vi "1d.vi"(6 "data in":T2={"Total counts"=0, "cps"=0.0, "live time"=0.0, "pulser"=0.0, "rare counts"=0.0, "other counts"=0.0, "total run time(sec)"=0.0, "adjusted run time(sec)"=0.0, "17O average"=1.0, "17O current"=1.0}, 8 "error in":errorcluster, 9 "1d state control":T3) -> (2 "MCA Histograms":u32[](graph), 4 "data out":T2={"Total counts"=0, "cps"=0.0, "live time"=0.0, "pulser"=0.0, "rare counts"=0.0, "other counts"=0.0, "total run time(sec)"=0.0, "adjusted run time(sec)"=0.0, "17O average"=1.0, "17O current"=1.0})   [LabVIEW 2016]
doc: "uses gated region to gather and parse 1d data"
uses:
  controls/1d/1d state event control.ctl
  spectrum/controls/count control.ctl
  Drivers/Pixie4DLL.dll
panel:
  out "Run time [s]":dbl
  out "number of events":dbl
  out "run data output":T1
  out "time":dbl
  out "counts":dbl
  in  "time for each slice(ms)":i32=100
  out "cps (slice)":dbl
  out "Pixie4DLL calls error":errorcluster
  out "run time":sgl
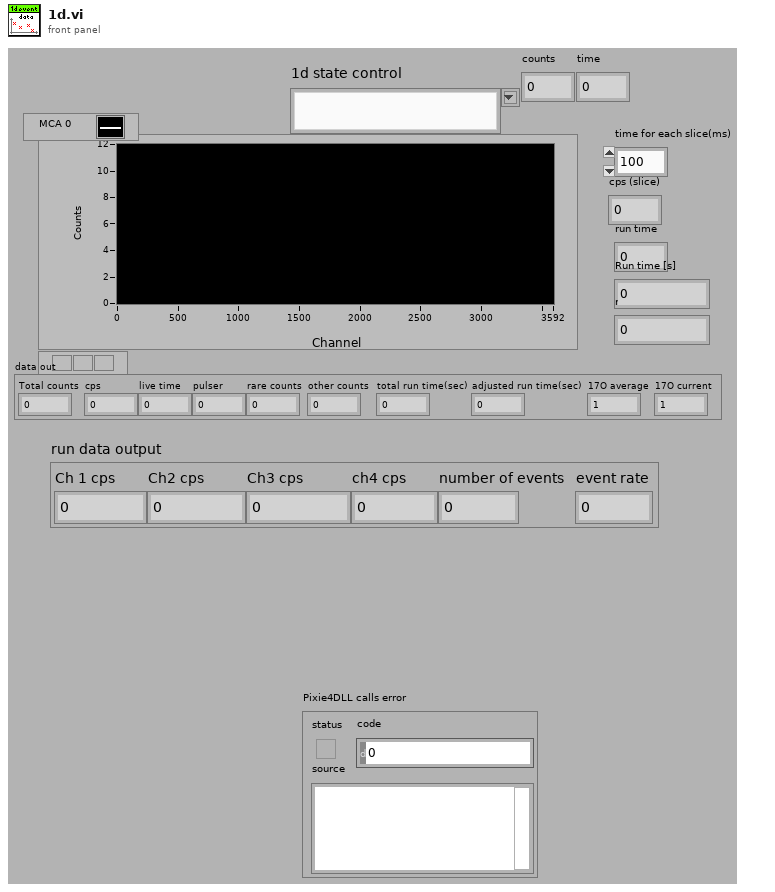
[diagram p1: front panel]
types:
  T1 = cluster{"Ch 1 cps":dbl, "Ch2 cps":dbl, "Ch3 cps":dbl, "ch4 cps":dbl, "number of events":dbl, "event rate":dbl}
  T2 = typedef "count control.ctl" = cluster{"Total counts":u32, "cps":dbl, "live time":dbl, "pulser":dbl, "rare counts":dbl, "other counts":dbl, "total run time(sec)":dbl, "adjusted run time(sec)":dbl, "17O average":dbl, "17O current":dbl}
  T3 = typedef "1d state event control.ctl" = string
  T4 = cluster{"input count rate 0":dbl, "input count rate 1":dbl, "input count rate 2":dbl, "input count rate 3":dbl, "number of events":dbl, "event rate":dbl}
  T5 = typedef "LVPoint32TypeDef.ctl" = cluster{"Horizontal":i32, "Vertical":i32}
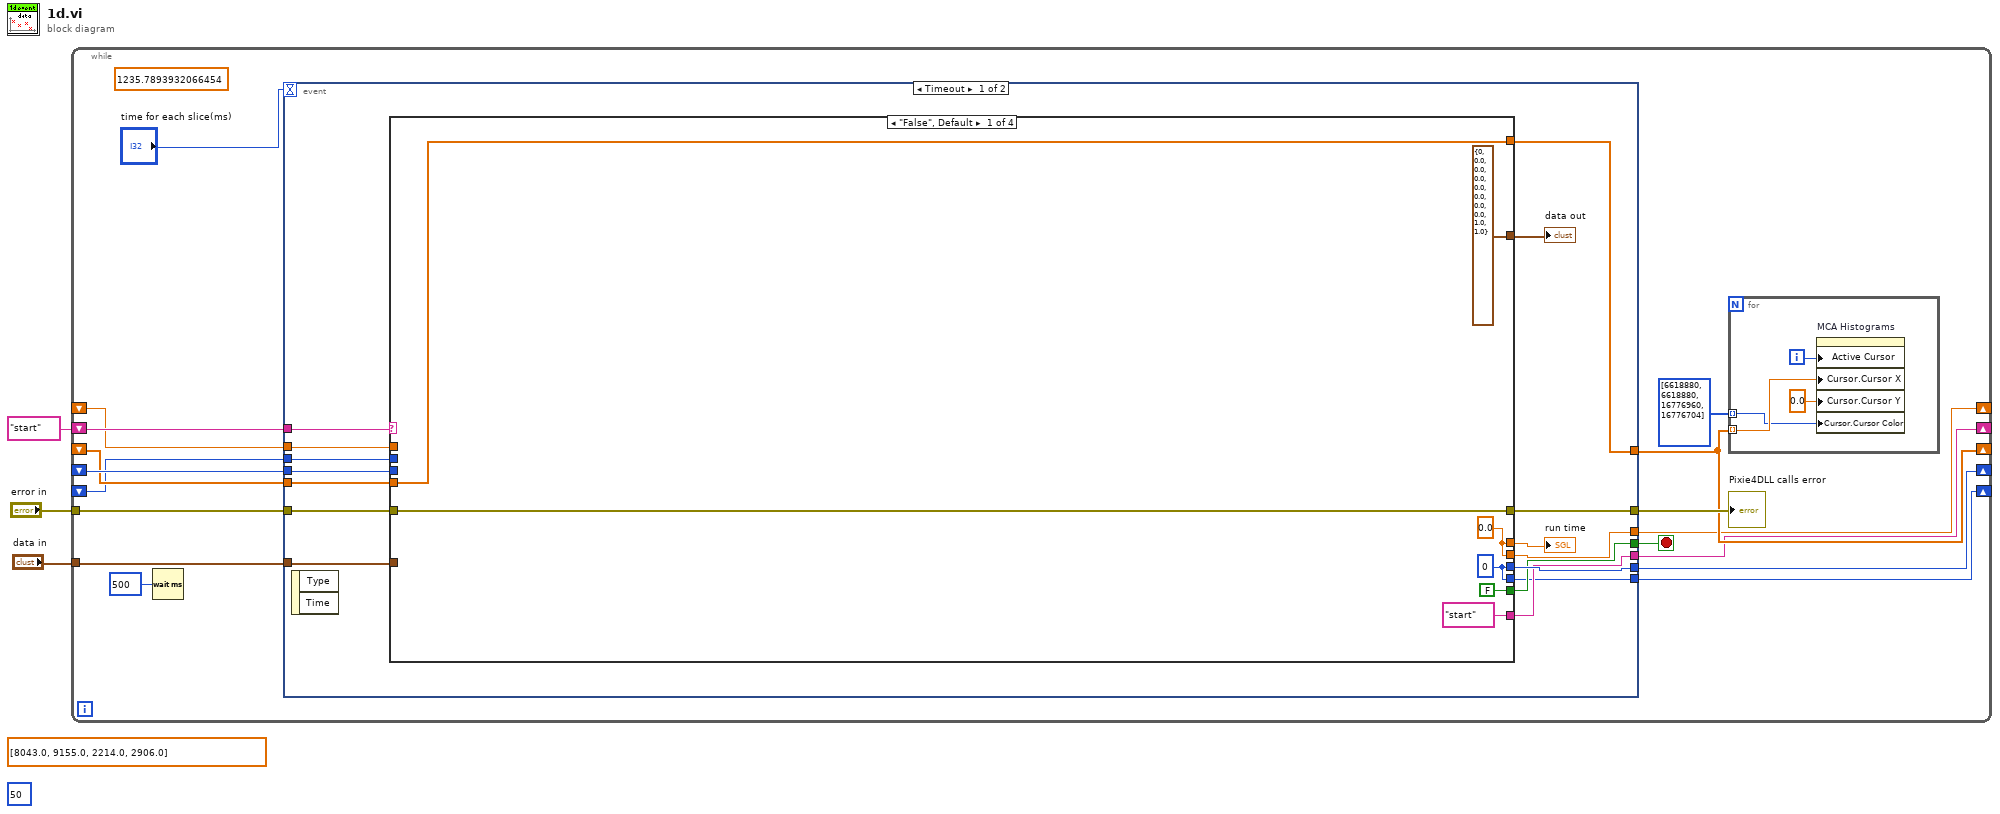
[diagram p0: block diagram]
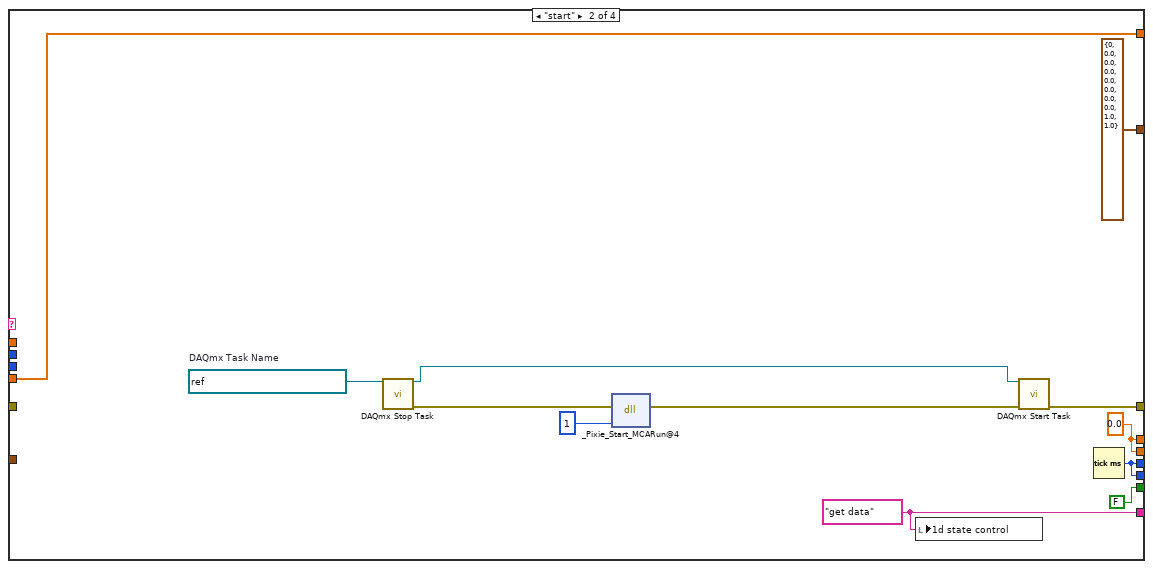
[diagram p2: hidden frame]
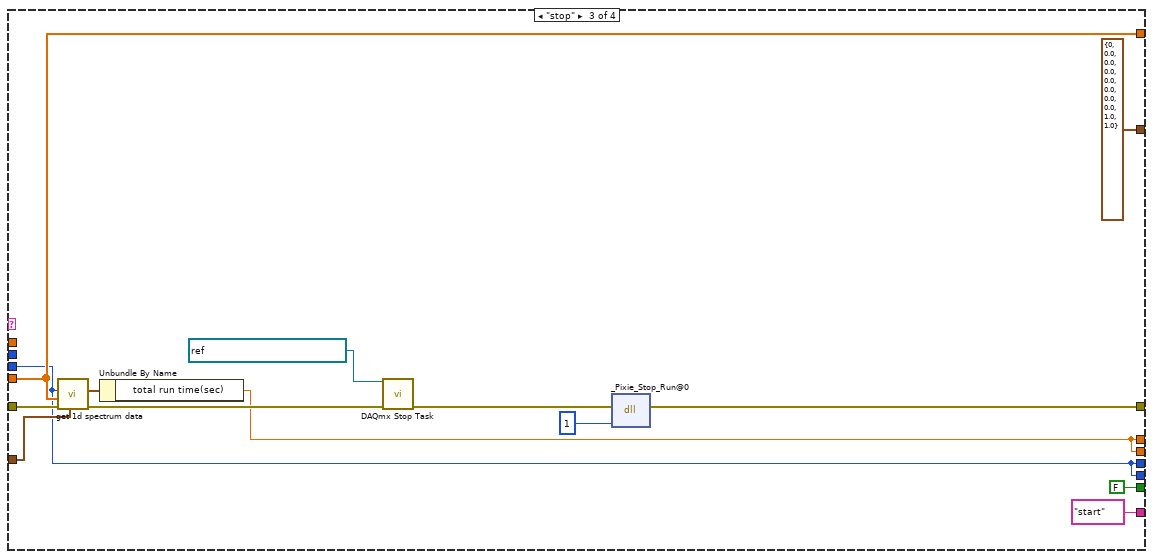
[diagram p3: hidden frame]
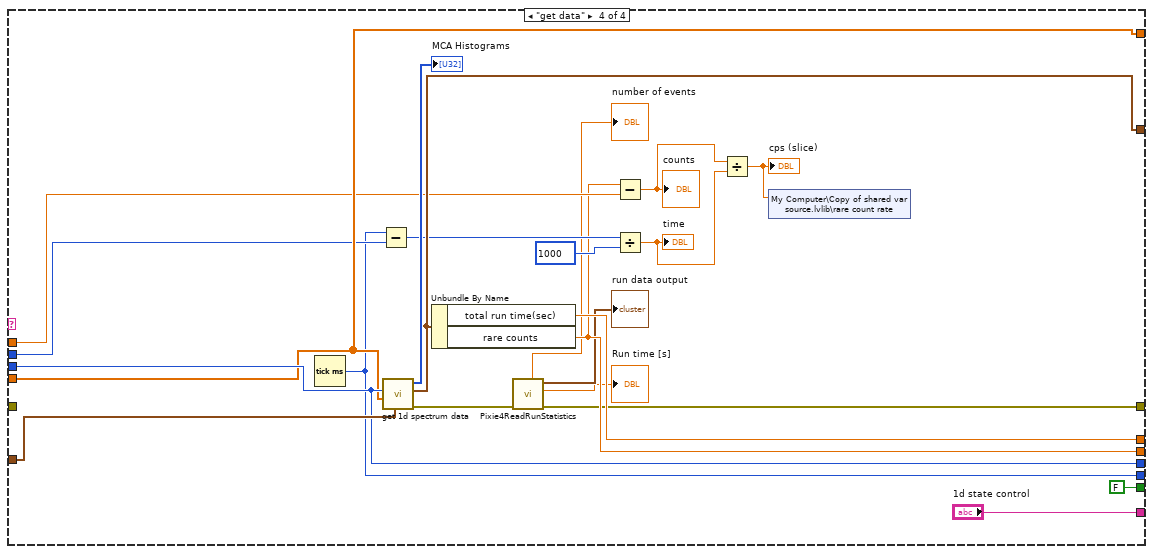
[diagram p4: hidden frame]
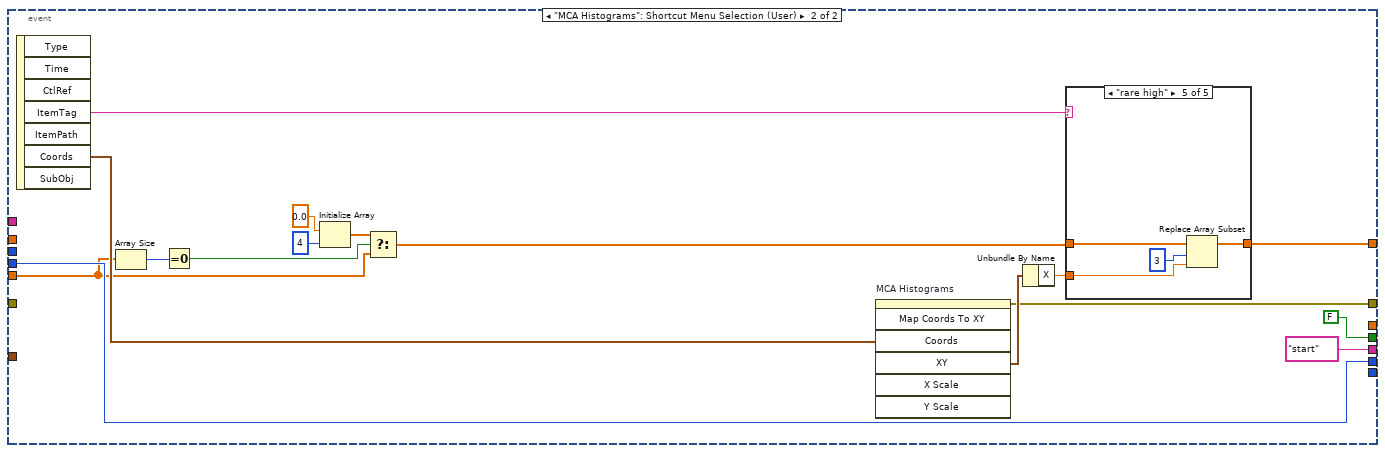
[diagram p5: hidden frame]
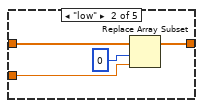
[diagram p7: hidden frame]
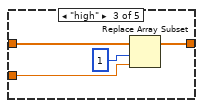
[diagram p8: hidden frame]
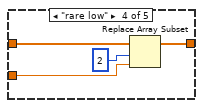
[diagram p9: hidden frame]
diagram:
  (unwired) dbl[] [8043.0, 9155.0, 2214.0, 2906.0] ("Array 2")
  (unwired) 50
  n1 = while {
    tunnel: "error in" -> [w18]
    tunnel: "data in" -> [w17]
    shift-right: [w16] -> _
    shift-left: _ -> [w20]
    shift-right: [w11] -> _
    shift-left: _ -> [w19]
    shift-right: [w8] -> _
    shift-left: T3 "start" ("1d state control") -> [w14]
    shift-right: [w7] -> _
    shift-left: _ -> [w6]
    shift-right: [w5] -> _
    shift-left: _ -> [w4]
    stop <- w13 stop-if-true
    (unwired) 1235.7893932066454 ("element")
    n2 = Wait (ms)(milliseconds to wait=u32 500) -> ()  [unwired: 1 out]
    n3 = event shown="[0] Timeout" {
      selector: _ -> [_ _]
      dyn-events: _ -> [_ _]
      timeout: "time for each slice(ms)" -> [_ _]
      tunnel: w20 -> [w40 w111]
      tunnel: w19 -> [w38 w100]
      tunnel: w18 -> [w37 _]
      tunnel: w17 -> [w36 _]
      tunnel: [w35 w111] -> w16
      tunnel: [w34 w106] -> w11
      tunnel: w14 -> [w33 _]
      tunnel: [w30 FALSE ("stop")] -> w13
      tunnel: [w32 w97] -> w12
      tunnel: [w29 T3 "start" ("1d state control")] -> w8
      tunnel: [w28 _] -> w7
      tunnel: w6 -> [w27 _]
      tunnel: [w26 _] -> w5
      tunnel: w4 -> [w25 _]
      event Timeout {
        n4 = event-data() -> ()  [unwired: 1 in, 2 out]
        n5 = case shown="\"False\", Default" w33 {
          tunnel: w40 -> [_ _ w61 w91]
          tunnel: [w41 w48 w60 w94] -> w39
          tunnel: w38 -> [w47 w58 w62 w88]
          tunnel: [T2 {"Total counts"=0, "cps"=0.0, "live time"=0.0, "pulser"=0.0, "rare counts"=0.0, "other counts"=0.0, "total run time(sec)"=0.0, "adjusted run time(sec)"=0.0, "17O average"=1.0, "17O current"=1.0} ("data in") T2 {"Total counts"=0, "cps"=0.0, "live time"=0.0, "pulser"=0.0, "rare counts"=0.0, "other counts"=0.0, "total run time(sec)"=0.0, "adjusted run time(sec)"=0.0, "17O average"=1.0, "17O current"=1.0} ("data in") T2 {"Total counts"=0, "cps"=0.0, "live time"=0.0, "pulser"=0.0, "rare counts"=0.0, "other counts"=0.0, "total run time(sec)"=0.0, "adjusted run time(sec)"=0.0, "17O average"=1.0, "17O current"=1.0} ("data in") w93] -> w31
          tunnel: w37 -> [w46 _ w72 _]
          tunnel: w36 -> [_ _ w71 w92]
          tunnel: [w42 w49 w61 w91] -> w35
          tunnel: [w47 w58 w62 w88] -> w34
          tunnel: [w46 w51 w65 w77] -> w32
          tunnel: [FALSE ("stop") FALSE ("stop") FALSE ("stop") FALSE ("stop")] -> w30
          tunnel: [T3 "start" ("1d state control") w55 T3 "start" ("1d state control") "1d state control"] -> w29
          tunnel: [w42 w49 w61 w79] -> w28
          tunnel: w27 -> [_ _ _ w87]
          tunnel: [w41 w48 w60 w81] -> w26
          tunnel: w25 -> [_ _ _ w82]
          frame "False", Default {
            w42 = u32 0 ("millisecond timer value")
            w41 = 0.0
          }
          frame "start" {
            w54 = refnum<k21> "MyCountEdgesTask"  # DAQmx Task Name
            w55 = T3 "get data" ("1d state control")
            w48 = 0.0
            n6 = call <vilib>:"DAQmx Stop Task.vi"("task/channels in"=w54) -> ("task out"=w50:refnum<k21>, "error out"=w53:errorcluster)  [unwired: 13 in]
            n7 = dll-call lib="D:/Users/wymanm/Desktop/DAQuiri - 2017a/PRIME DAQ 2017a/Drivers/Pixie4DLL.dll" fn="_Pixie_Start_MCARun@4"(error in=w53, "mode"=u16 1 ("ModNum")) -> (error out=w52:errorcluster)  [unwired: 4 in, 1 out]
            n8 = local write "1d state control"(w55) -> ()
            n9 = call <vilib>:"DAQmx Start Task.vi"("task/channels in"=w50, "error in"=w52) -> ("error out"=w51:errorcluster)  [unwired: 12 in, 1 out]
            n10 = Tick Count (ms)() -> (millisecond timer value=w49:u32)
          }
          frame "stop" {
            n11 = call "get 1d spectrum data.vi"("data in"=w71, "error in"=w72, "gates"=w62, "time in"=w61) -> ("error out 2"=w67:errorcluster, "data out"=w64:T2)  [unwired: 3 in, 3 out]
            n12 = Unbundle By Name(w64) -> ("total run time(sec)"=w60:dbl)
            n13 = call <vilib>:"DAQmx Stop Task.vi"("task/channels in"=refnum<k21> "MyCountEdgesTask", "error in"=w67) -> ("error out"=w66:errorcluster)  [unwired: 12 in, 1 out]
            n14 = dll-call lib="D:/Users/wymanm/Desktop/DAQuiri - 2017a/PRIME DAQ 2017a/Drivers/Pixie4DLL.dll" fn="_Pixie_Stop_Run@0"(error in=w66, "mode"=u16 1 ("ModNum")) -> (error out=w65:errorcluster)  [unwired: 4 in, 1 out]
          }
          frame "get data" {
            n15 = Tick Count (ms)() -> (millisecond timer value=w79:u32)
            n16 = Subtract(x=w79, y=w87) -> (x-y=w86:u32)
            n17 = call "get 1d spectrum data.vi"("data in"=w92, "gates"=w88, "time in"=w91) -> ("error out 2"=w78:errorcluster, "data out"=w93:T2, "MCA Histograms"=→"MCA Histograms":u32[])  [unwired: 4 in, 2 out]
            n18 = Unbundle By Name(w93) -> ("total run time(sec)"=w94:dbl, "rare counts"=w81:dbl)
            n19 = call "Pixie4ReadRunStatistics.vi"("error in (no error)"=w78) -> ("error out"=w77:errorcluster, "Run time [s]"=→"Run time [s]":dbl, "run data output"=→"run data output":T4, "number of events"=→"number of events":dbl)  [unwired: 7 in]
            n20 = Subtract(x=w81, y=w82) -> (x-y=w80:dbl)
            "counts" <- w80
            n21 = Divide(x=w86, y=u32 1000) -> (x/y=w84:dbl)
            "time" <- w84
            n22 = Divide(x=w80, y=w84) -> (x/y=w83:dbl)
            "cps (slice)" <- w83
            n23 = shared-variable "My Computer\\Copy of shared var source.lvlib\\rare count rate"(w83) -> ()  [unwired: 1 in, 1 out]
          }
        }
        "run time" <- w39
        "data out" <- w31
      }
      event "MCA Histograms": Shortcut Menu Selection (User) {
        n24 = event-data() -> ("ItemTag"=w110:string, "Coords"=w109:T5)  [unwired: 1 in, 5 out]
        n25 = Array Size(array=w100) -> (size(s)=w103:i32)
        n26 = Equal To 0?(x=w103) -> (x = 0?=w102:bool)
        n27 = Initialize Array(0.0 ("element"), 4 ("dimension size")) -> (w101:dbl[])
        n28 = Select(t=w101, s=w102, f=w100) -> (s? t:f=w99:dbl[])
        n29 = invoke on="MCA Histograms" class="WFGraph (strict)" method="Map Coords To XY"("Coords"=w109) -> (error out=w97:errorcluster, "XY"=w108:cluster{"X":dbl, "Y":dbl})  [unwired: 6 in, 5 out]
        n30 = Unbundle By Name(w108) -> ("X"=w107:dbl)
        n31 = case shown="\"rare high\"" w110 {
          tunnel: w99 -> [w112 w116 w120 w124 w128]
          tunnel: w107 -> [_ w115 w119 w123 w127]
          tunnel: [w112 w113 w117 w121 w125] -> w106
          frame "False", Default {
          }
          frame "low" {
            n32 = Replace Array Subset(array=w116, new element=w115, index=0) -> (w113:dbl[])
          }
          frame "high" {
            n33 = Replace Array Subset(array=w120, new element=w119, index=1) -> (w117:dbl[])
          }
          frame "rare low" {
            n34 = Replace Array Subset(array=w124, new element=w123, index=2) -> (w121:dbl[])
          }
          frame "rare high" {
            n35 = Replace Array Subset(array=w128, new element=w127, index=3) -> (w125:dbl[])
          }
        }
      }
    }
    "Pixie4DLL calls error" <- w12
    n36 = for {
      tunnel: w11 -> [w24] mode=indexing
      tunnel: u32[] [6618880, 6618880, 16776960, 16776704] ("Array 2") -> [w21] mode=indexing
      i -> [w23]
      n37 = property on="MCA Histograms" class="WFGraph (strict)"("Active Cursor"=w23, "Cursor.Cursor X"=w24, "Cursor.Cursor Y"=0.0 ("Cursor.Cursor Position:Cursor Y"), "Cursor.Cursor Color"=w21) -> ()  [unwired: 2 in, 2 out]
    }
  }
